vi "test - restore variable value.vi"(8 "error in (no error)":errorcluster, 11 "TestCase in":refnum<class "csm-ini-variable-addon.lvclass">) -> (0 "error out":errorcluster, 3 "TestCase out":refnum<class "csm-ini-variable-addon.lvclass">)   [LabVIEW 2017, in "csm-ini-variable-addon.lvclass"]
uses:
  csm-ini-variable-addon.lvclass
  819d10de-cc93-4901-8476-a53ff0da62fe.vi
  170bfbe0-d683-4dc2-8150-79f99a429e18.vi
  d36187ab-fd98-4cab-9202-c0bc5d57495a.vi
  4331c652-d221-4445-b443-08c445718bf9.vi
  c7eb524b-4dac-4139-8eef-18ef3fc17f72.vi
  d8318c36-89ae-4345-a8d4-853983db99ea.vi
  70612327-44ab-4a02-9772-ce9fbf697da7.vi
  819d10de-cc93-4901-8476-a53ff0da62fe.vi/b09b9099-6be0-413b-8afc-4908471460c3.vi
  INI-Static-Variable-Support/_Support/FlagInstance-CSMINIVariable.vi
  170bfbe0-d683-4dc2-8150-79f99a429e18.vi/99de0c97-112a-4c86-9094-c187659127e1.vi
  <vilib>/Utility/error.llb/Clear Errors.vi
  d36187ab-fd98-4cab-9202-c0bc5d57495a.vi/b09b9099-6be0-413b-8afc-4908471460c3.vi
  4331c652-d221-4445-b443-08c445718bf9.vi/b09b9099-6be0-413b-8afc-4908471460c3.vi
  c7eb524b-4dac-4139-8eef-18ef3fc17f72.vi/99de0c97-112a-4c86-9094-c187659127e1.vi
  d8318c36-89ae-4345-a8d4-853983db99ea.vi/b09b9099-6be0-413b-8afc-4908471460c3.vi
  70612327-44ab-4a02-9772-ce9fbf697da7.vi/b09b9099-6be0-413b-8afc-4908471460c3.vi
  <userlib>/_NEVSTOP/Communicable State Machine(CSM)/_Support/ChangeFlag/ChangeFlag-Read.vi
  <userlib>/_NEVSTOP/Communicable State Machine(CSM)/_Support/ChangeFlag/ChangeFlagDB.vi
  <vilib>/Utility/Data Type/Get Type Information.vi
  <userlib>/_NEVSTOP/Communicable State Machine(CSM)/addons/API-String-Arugments-Support/_Support/Data To SingleElementsArray_csm.vi
  INI-Static-Variable-Support/_Support/Parse Used Session and Name.vi
  <userlib>/_NEVSTOP/Communicable State Machine(CSM)/addons/API-String-Arugments-Support/_Support/Data To API String Arguments.vi
  INI-Static-Variable-Support/_Support/INI-FGV(lvlibp).vi
  INI-Static-Variable-Support/_Support/Populate String with INI Variable.vi
  <userlib>/_NEVSTOP/Communicable State Machine(CSM)/addons/API-String-Arugments-Support/_Support/Convert API String Arguments to Data(variant).vi
  <userlib>/_NEVSTOP/Communicable State Machine(CSM)/addons/API-String-Arugments-Support/_Support/SingleElementsArray To Data_csm.vi
  INI-Static-Variable-Support/INI-Static-Variable-Support.lvlib
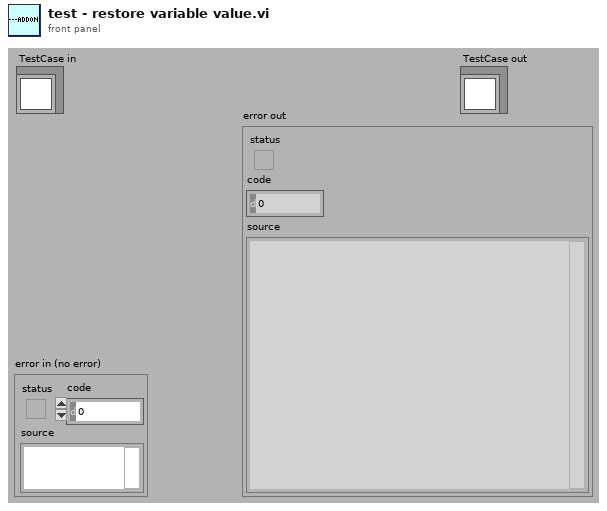
[diagram p1: front panel]
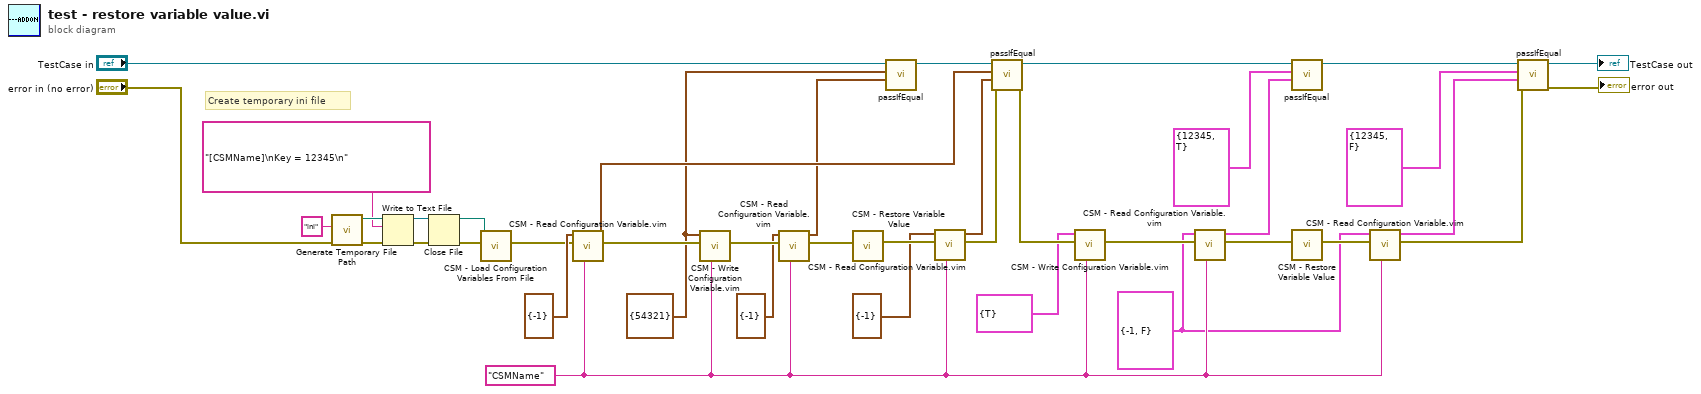
[diagram p0: block diagram]
diagram:
  w7 = cluster{"Key":i32, "Boolean":bool} {"Key"=-1, "Boolean"=FALSE}
  w18 = cluster{"Key":i32} {"Key"=54321}
  w8 = "CSMName" ("Section Name(\"\" as Default)")
  # "Create temporary ini file"
  n1 = call <vilib>:"Generate Temporary File Path.vi"("error in (no error)"="error in (no error)", "Temporary File Extension (tmp)"="ini") -> ("error out"=w39:errorcluster, "Unique Temporary File Path"=w36:path)  [unwired: 8 in]
  n2 = Write to Text File(file (use dialog)=w36, text="[CSMName]\nKey = 12345\n", error in=w39) -> (refnum out=w35:refnum<file>, error out=w37:errorcluster)  [unwired: 1 in, 1 out]
  n3 = Close File(refnum=w35, error in=w37) -> (path=w32:path, error out=w34:errorcluster)
  n4 = call "CSM - Load Configuration Variables From File.vi"("error in (no error)"=w34, "Path"=w32) -> ("error out"=w29:errorcluster)  [unwired: 7 in]
  n5 = call "CSM - Read Configuration Variable.vim"("Section Name(\"\" as Default)"=w8, "error in (no error)"=w29, "config prototype(Cluster Prefered)"=cluster{"Key":i32} {"Key"=-1}) -> ("error out"=w25:errorcluster, "config out"=w27:cluster{"Key":i32})  [unwired: 5 in]
  n6 = call "CSM - Write Configuration Variable.vim"("Section Name(\"\" as Default)"=w8, "error in (no error)"=w25, "Variant"=w18) -> ("error out"=w23:errorcluster)  [unwired: 5 in, 1 out]
  n7 = call "CSM - Read Configuration Variable.vim"("Section Name(\"\" as Default)"=w8, "error in (no error)"=w23, "config prototype(Cluster Prefered)"=cluster{"Key":i32} {"Key"=-1}) -> ("error out"=w22:errorcluster, "config out"=w17:cluster{"Key":i32})  [unwired: 5 in]
  n8 = call "CSM - Restore Variable Value.vi"("error in (no error)"=w22) -> ("error out"=w28:errorcluster)  [unwired: 8 in]
  n9 = call-dynamic "passIfEqual.vi"("y"=w17, "x"=w18, "TestCase in"="TestCase in") -> ("TestCase out"=w19:refnum<class "csm-ini-variable-addon.lvclass">)  [unwired: 7 in, 1 out]
  n10 = call "CSM - Read Configuration Variable.vim"("Section Name(\"\" as Default)"=w8, "error in (no error)"=w28, "config prototype(Cluster Prefered)"=cluster{"Key":i32} {"Key"=-1}) -> ("error out"=w30:errorcluster, "config out"=w26:cluster{"Key":i32})  [unwired: 5 in]
  n11 = call-dynamic "passIfEqual.vi"("error in (no error)"=w30, "y"=w26, "x"=w27, "TestCase in"=w19) -> ("error out"=w16:errorcluster, "TestCase out"=w13:refnum<class "csm-ini-variable-addon.lvclass">)  [unwired: 6 in]
  n12 = call "CSM - Write Configuration Variable.vim"("Section Name(\"\" as Default)"=w8, "error in (no error)"=w16, "Variant"=cluster{"Boolean":bool} {"Boolean"=TRUE}) -> ("error out"=w15:errorcluster)  [unwired: 5 in, 1 out]
  n13 = call "CSM - Read Configuration Variable.vim"("Section Name(\"\" as Default)"=w8, "error in (no error)"=w15, "config prototype(Cluster Prefered)"=w7) -> ("error out"=w10:errorcluster, "config out"=w12:cluster{"Key":i32, "Boolean":bool})  [unwired: 5 in]
  n14 = call-dynamic "passIfEqual.vi"("y"=w12, "x"=cluster{"Key":i32, "Boolean":bool} {"Key"=12345, "Boolean"=TRUE}, "TestCase in"=w13) -> ("TestCase out"=w6:refnum<class "csm-ini-variable-addon.lvclass">)  [unwired: 7 in, 1 out]
  n15 = call "CSM - Restore Variable Value.vi"("error in (no error)"=w10) -> ("error out"=w9:errorcluster)  [unwired: 8 in]
  n16 = call "CSM - Read Configuration Variable.vim"("Section Name(\"\" as Default)"=w8, "error in (no error)"=w9, "config prototype(Cluster Prefered)"=w7) -> ("error out"=w5:errorcluster, "config out"=w1:cluster{"Key":i32, "Boolean":bool})  [unwired: 5 in]
  n17 = call-dynamic "passIfEqual.vi"("error in (no error)"=w5, "y"=w1, "x"=cluster{"Key":i32, "Boolean":bool} {"Key"=12345, "Boolean"=FALSE}, "TestCase in"=w6) -> ("error out"=→"error out":errorcluster, "TestCase out"=→"TestCase out":refnum<class "csm-ini-variable-addon.lvclass">)  [unwired: 6 in]
